vi "ATM.vi"() -> ()   [LabVIEW 2025]
uses:
  Controls/States.ctl
panel:
  in  "Enter":bool
  in  "User Input":string
  in  "Right Buttons":T1
  out "Right Menu":T2
  in  "Left Buttons":T1
  out "Left Menu":T2
  in  "Card Simulator":bool
  out "ATM Messages":string
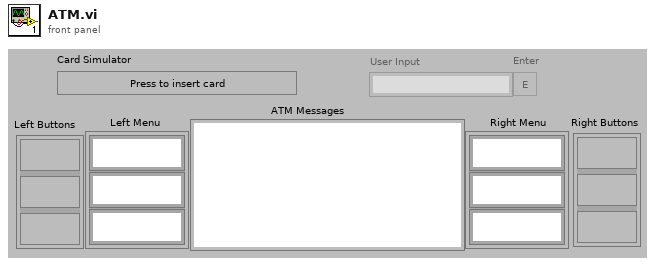
[diagram p1: front panel]
types:
  T1 = cluster{"Func Button":bool, "Func Button 2":bool, "Func Button 3":bool}
  T2 = cluster{"RFS String":string, "RFS String 2":string, "RFS String 3":string}
  T3 = typedef "States.ctl" = enum16{"Initialization", "Waiting For Instruction", "Card Inserted", "Identification", "Balance", "Deposit Message", "Deposit Complete", "Withdraw Message", "Withdraw Possible?", "Withdraw Complete", "Withdraw Failed", "Fast Cash", "Shutdown"}
  T4 = cluster{"Enter":refnum<vi>, "User Input":refnum<vi>, "Right Buttons":refnum<vi>, "Left Buttons":refnum<vi>, "Card Simulator":refnum<vi>, "Right Menu":refnum<vi>, "Left Menu":refnum<vi>, "ATM Messages":refnum<vi>}
  T5 = enum8{"Enabled", "Disabled", "Disabled and Grayed Out"}
  T6 = enum16{"Welcome", "Main Menu", "Account Verif Failed", "Session Terminate", "Deposit", "Deposit complete", "Withdrawal", "Withdrawal complete", "Withdrawal failed", "Balance Inquiry"}
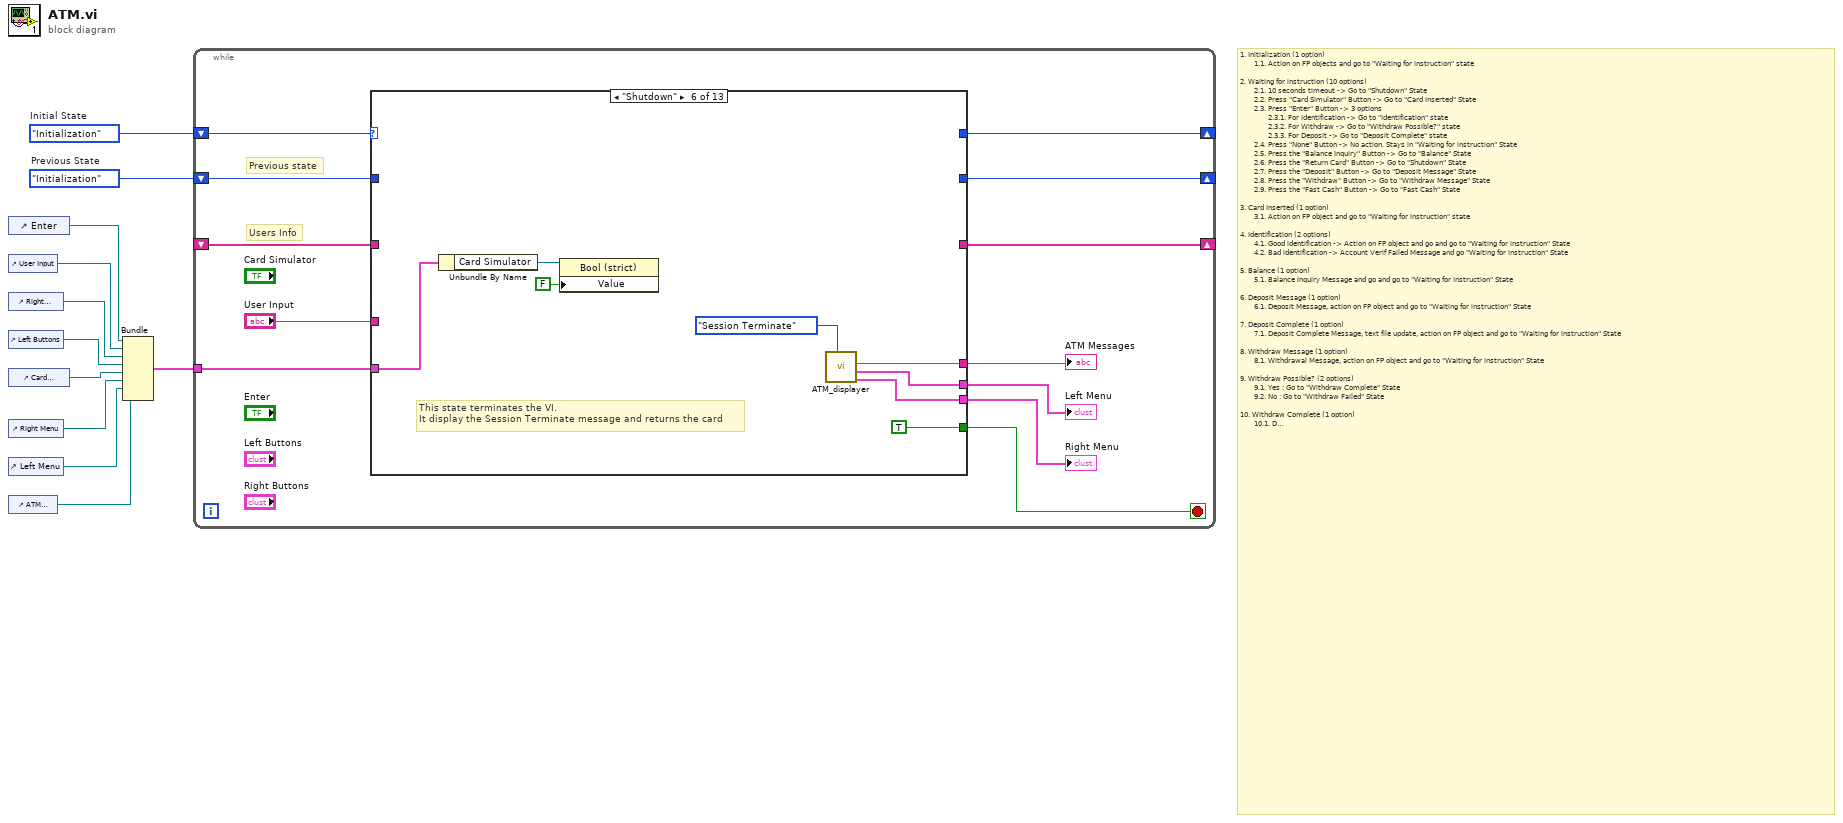
[diagram p0: block diagram]
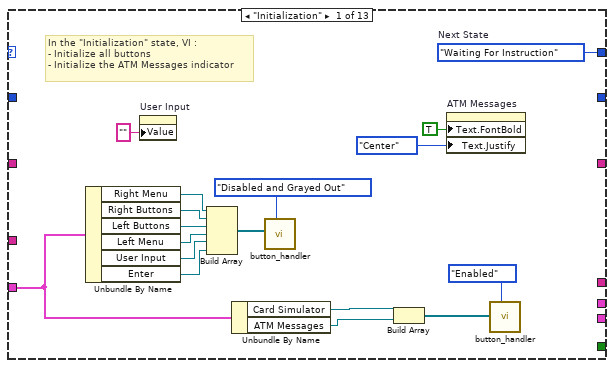
[diagram p2: hidden frame]
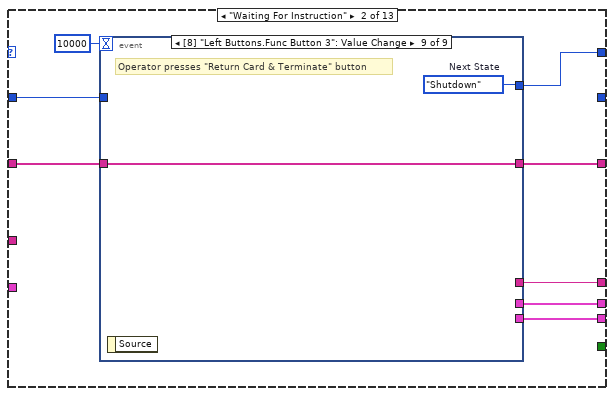
[diagram p3: hidden frame]
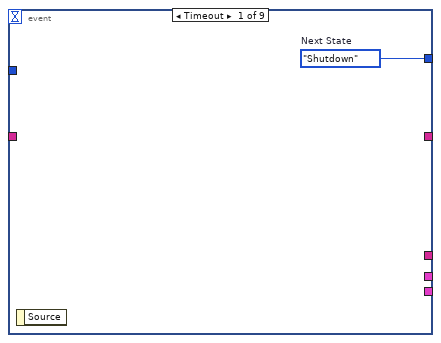
[diagram p4: hidden frame]
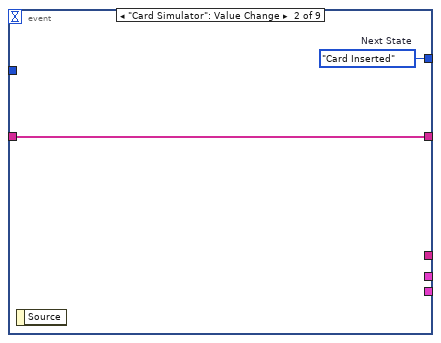
[diagram p5: hidden frame]
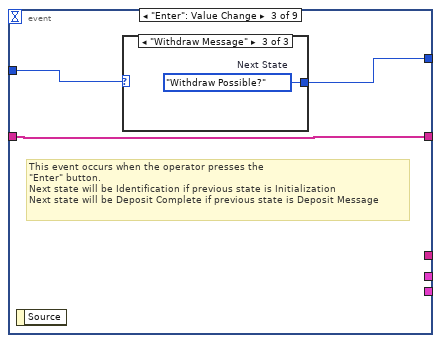
[diagram p6: hidden frame]
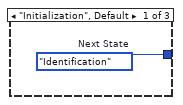
[diagram p7: hidden frame]
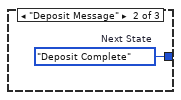
[diagram p8: hidden frame]
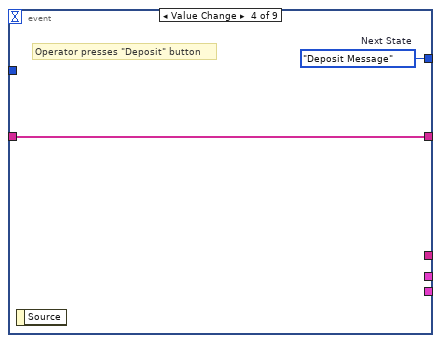
[diagram p9: hidden frame]
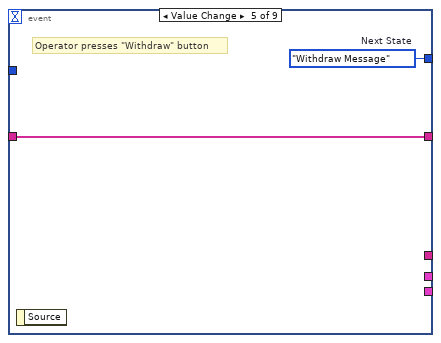
[diagram p10: hidden frame]
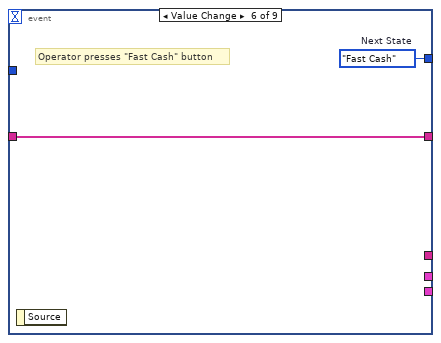
[diagram p11: hidden frame]
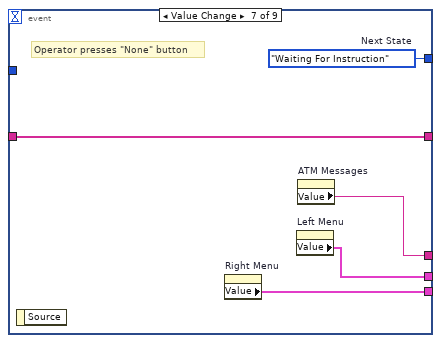
[diagram p12: hidden frame]
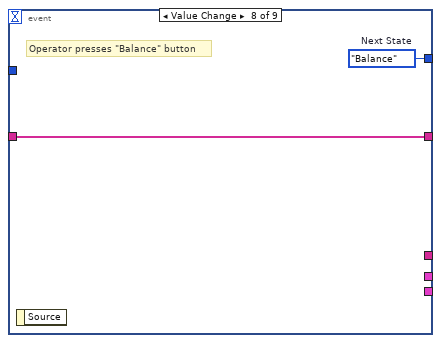
[diagram p13: hidden frame]
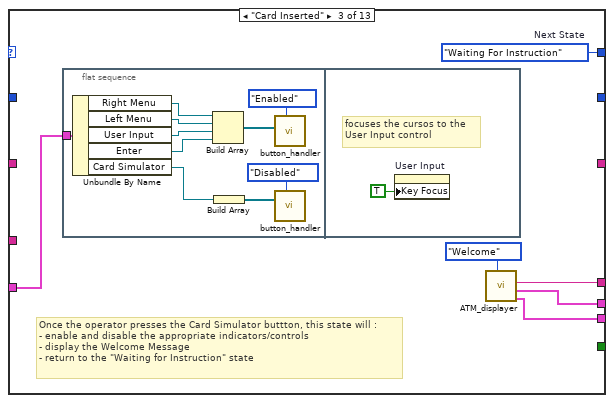
[diagram p14: hidden frame]
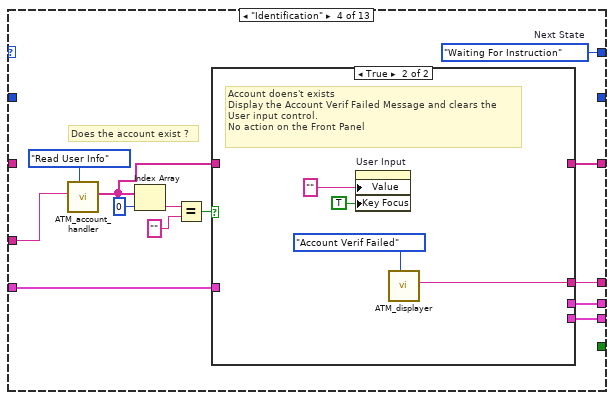
[diagram p15: hidden frame]
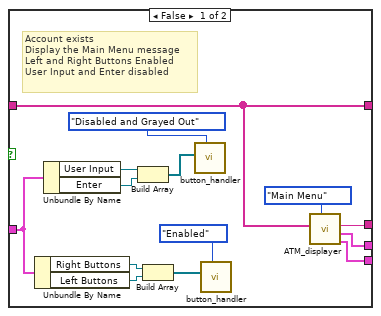
[diagram p16: hidden frame]
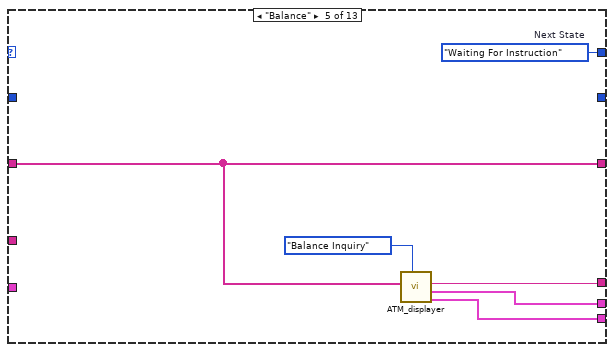
[diagram p17: hidden frame]
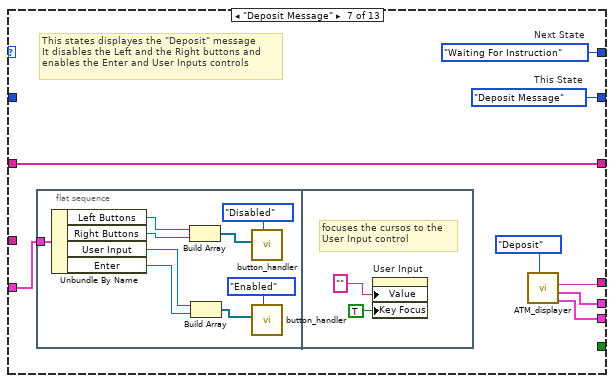
[diagram p18: hidden frame]
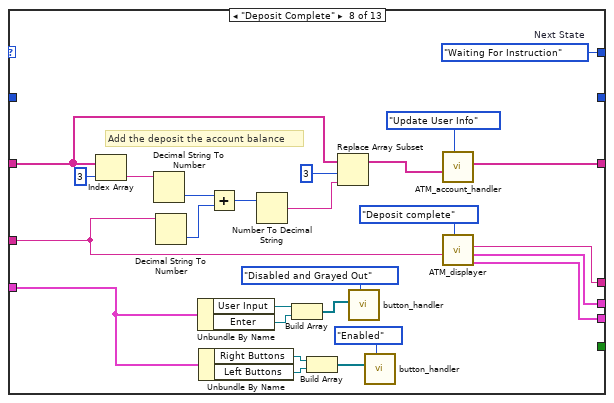
[diagram p19: hidden frame]
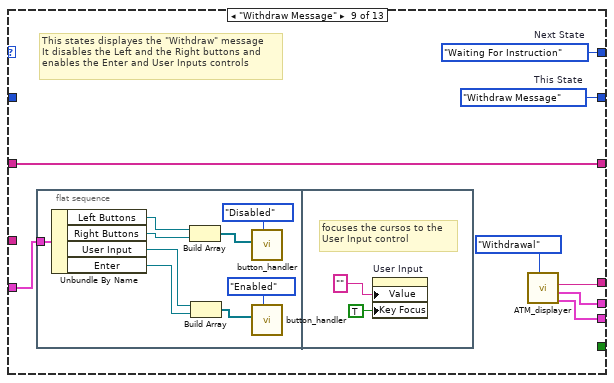
[diagram p20: hidden frame]
diagram:
  w1 = States."Initialization"  # Previous State
  w11 = States."Initialization"  # Initial State
  # "1. Initialization (1 option)\n       1.1. Action on FP objects and go to \"Waiting for instruction\" state\n\n2. Waiting for instruction (10 options)\n       2.1. 10 seconds timeout -> Go to \"Shutdown\" State\n       2.2. Press \"Card Simulator\" Button -> Go to \"Card Inserted\" State\n       2.3. Press \"Enter\" Button -> 3 options\n              2.3.1. For identification -> Go to \"Identification\" state  \n              2.3.2. For Withdraw -> Go to \"Withdraw Possible?\" state\n              2.3.3. For Deposit -> Go to \"Deposit Complete\" state\n       2.4. Press \"None\" Button -> No action. Stays in \"Waiting for instruction\" State\n       2.5. Press the \"Balance Inquiry\" Button -> Go to \"Balance\" State\n       2.6. Press the \"Return Card\" Button -> Go to \"Shutdown\" State\n       2.7. Press the \"Deposit\" Button -> Go to \"Deposit Message\" State\n       2.8. Press the \"Withdraw\" Button -> Go to \"Withdraw Message\" State\n       2.9. Press the \"Fast Cash\" Button -> Go to \"Fast Cash\" State\n\n3. Card Inserted (1 option)\n       3.1. Action on FP object and go to \"Waiting for instruction\" state\n\n4. Identification (2 options)\n       4.1. Good identification -> Action on FP object and go and go to \"Waiting for instruction\" State\n       4.2. Bad identification -> Account Verif Failed Message and go \"Waiting for instruction\" State\n\n5. Balance (1 option)\n       5.1. Balance Inquiry Message and go and go to \"Waiting for instruction\" State\n\n6. Deposit Message (1 option)\n       6.1. Deposit Message, action on FP object and go to \"Waiting for instruction\" State\n\n7. Deposit Complete (1 option)\n       7.1. Deposit Complete Message, text file update, action on FP object and go to \"Waiting for instruction\" State\n\n8. Withdraw Message (1 option)\n       8.1. Withdrawal Message, action on FP object and go to \"Waiting for instruction\" State\n\n9. Withdraw Possible? (2 options)\n       9.1. Yes : Go to \"Withdraw Complete\" State\n       9.2. No : Go to \"Withdraw Failed\" State\n\n10. Withdraw Complete (1 option)\n       10.1. Deposit Complete Message, text file update, action on FP object and go to \"Waiting for instructio\n\n11. Withdraw Failed (1 option)\n       11.1. Withdrawal Failed Message, action on FP object and go to \"Waiting for instructio\n\n12. Fast Cash (1 option)\n       12.1. Go to \"Withdrawal Possible?\" State\n\n13. Shutdown (1 option)\n       13.1. Session Terminate Message and Terminate Program"
  n1 = control-ref of="Enter"() -> (w10:refnum<vi>)
  n2 = control-ref of="User Input"() -> (w9:refnum<vi>)
  n3 = control-ref of="Right Buttons"() -> (w8:refnum<vi>)
  n4 = control-ref of="Left Buttons"() -> (w7:refnum<vi>)
  n5 = control-ref of="Card Simulator"() -> (w6:refnum<vi>)
  n6 = control-ref of="Right Menu"() -> (w5:refnum<vi>)
  n7 = control-ref of="Left Menu"() -> (w3:refnum<vi>)
  n8 = control-ref of="ATM Messages"() -> (w4:refnum<vi>)
  n9 = Bundle("Enter"=w10, "User Input"=w9, "Right Buttons"=w8, "Left Buttons"=w7, "Card Simulator"=w6, "Right Menu"=w5, "Left Menu"=w3, "ATM Messages"=w4) -> (w2:T4)  [unwired: 1 in]
  n10 = while {
    tunnel: w2 -> [w22]
    shift-right: [w21] -> _
    shift-left: w11 -> [w23]
    shift-right: [w15] -> _
    shift-left: _ -> [w14]
    shift-right: [w13] -> _
    shift-left: w1 -> [w12]
    stop <- w19 stop-if-true
    # "Previous state"
    # "Users Info"
    n11 = case shown="\"Shutdown\"" w23 {
      tunnel: w22 -> [w32 _ w73 w92 _ w129 w138 w156 w183 _ w230 w247 _]
      tunnel: [w25 w48 w75 w93 w123 _ w137 w176 w182 w199 w241 w256 w262] -> w21
      tunnel: [_ w46 w78 w96 w126 w133 w141 w154 w186 _ w229 w246 _] -> w20
      tunnel: [_ _ _ _ _ TRUE _ _ _ _ _ _ _] -> w19
      tunnel: [_ w45 w77 w95 w122 w132 w140 w179 w185 _ w244 w259 _] -> w18
      tunnel: [_ w44 w76 w94 w121 w131 w139 w178 w184 _ w243 w258 _] -> w17
      tunnel: "User Input" -> [_ _ _ w101 _ _ _ w155 _ w210 w223 _ _]
      tunnel: [_ w42 _ w90 w124 _ w136 w165 w181 w200 w239 w245 w261] -> w15
      tunnel: w14 -> [_ w43 _ _ w124 _ w136 w169 w181 w202 w228 w245 w261]
      tunnel: [_ _ _ _ _ _ w135 _ w180 w213 _ _ w260] -> w13
      tunnel: w12 -> [_ w41 _ _ _ _ _ _ _ w213 w226 _ _]
      frame "Initialization" {
        w25 = States."Waiting For Instruction"  # Next State
        # "In the \"Initialization\" state, VI :\n- Initialize all buttons\n- Initialize the ATM Messages indicator"
        n12 = Unbundle By Name(w32) -> ("Right Menu"=w40:refnum<vi>, "Right Buttons"=w39:refnum<vi>, "Left Buttons"=w38:refnum<vi>, "Left Menu"=w37:refnum<vi>, "User Input"=w36:refnum<vi>, "Enter"=w35:refnum<vi>)
        n13 = property on="User Input" class="Str"("Value"="" ("User Input")) -> ()  [unwired: 2 in, 2 out]
        n14 = Build Array(w40, w39, w38, w37, w36, w35) -> (w34:refnum<vi>[])
        n15 = Unbundle By Name(w32) -> ("Card Simulator"=w24:refnum<vi>, "ATM Messages"=w31:refnum<vi>)
        n16 = call "button_handler.vi"("Disabled"=T5."Disabled and Grayed Out", "reference"=w34) -> ()  [unwired: 10 in]
        n17 = Build Array(w24, w31) -> (w30:refnum<vi>[])
        n18 = property on="ATM Messages" class="Str"("Text.FontBold"=TRUE ("Text.Font:Bold"), "Text.Justify"=enum16{"Left", "Center", "Right"}."Center" ("Text.Justification")) -> ()  [unwired: 2 in, 2 out]
        n19 = call "button_handler.vi"("Disabled"=T5."Enabled", "reference"=w30) -> ()  [unwired: 10 in]
      }
      frame "Waiting For Instruction" {
        n20 = event shown="[8] \"Left Buttons.Func Button 3\": Value Change" {
          selector: _ -> [_ _ _ _ _ _ _ _ _]
          dyn-events: _ -> [_ _ _ _ _ _ _ _ _]
          timeout: 10000 -> [_ _ _ _ _ _ _ _ _]
          tunnel: [w49 w51 w54 w58 w60 w62 w68 w70 w72] -> w48
          tunnel: [_ _ _ _ _ _ w67 _ _] -> w46
          tunnel: [_ _ _ _ _ _ w66 _ _] -> w45
          tunnel: [_ _ _ _ _ _ w65 _ _] -> w44
          tunnel: w43 -> [_ w50 w53 w59 w61 w63 w64 w69 w71]
          tunnel: [_ w50 w53 w59 w61 w63 w64 w69 w71] -> w42
          tunnel: w41 -> [_ _ w52 _ _ _ _ _ _]
          event Timeout {
            w49 = States."Shutdown"  # Next State
            n21 = event-data() -> ()  [unwired: 1 in, 1 out]
          }
          event "Card Simulator": Value Change {
            w51 = States."Card Inserted"  # Next State
            n22 = event-data() -> ()  [unwired: 1 in, 1 out]
          }
          event "Enter": Value Change {
            # "This event occurs when the operator presses the\n\"Enter\" button.\nNext state will be Identification if previous state is Initialization\nNext state will be Deposit Complete if previous state is Deposit Message"
            n23 = event-data() -> ()  [unwired: 1 in, 1 out]
            n24 = case shown="\"Withdraw Message\"" w52 {
              tunnel: [w55 w56 w57] -> w54
              frame "Initialization", Default {
                w55 = States."Identification"  # Next State
              }
              frame "Deposit Message" {
                w56 = States."Deposit Complete"  # Next State
              }
              frame "Withdraw Message" {
                w57 = States."Withdraw Possible?"  # Next State
              }
            }
          }
          event "Right Buttons.Func Button": Value Change {
            w58 = States."Deposit Message"  # Next State
            # "Operator presses \"Deposit\" button"
            n25 = event-data() -> ()  [unwired: 1 in, 1 out]
          }
          event "Right Buttons.Func Button 2": Value Change {
            w60 = States."Withdraw Message"  # Next State
            # "Operator presses \"Withdraw\" button"
            n26 = event-data() -> ()  [unwired: 1 in, 1 out]
          }
          event "Right Buttons.Func Button 3": Value Change {
            w62 = States."Fast Cash"  # Next State
            # "Operator presses \"Fast Cash\" button"
            n27 = event-data() -> ()  [unwired: 1 in, 1 out]
          }
          event "Left Buttons.Func Button": Value Change {
            w68 = States."Waiting For Instruction"  # Next State
            # "Operator presses \"None\" button"
            n28 = event-data() -> ()  [unwired: 1 in, 1 out]
            n29 = property on="Right Menu" class="Clust (strict)"() -> ("Value"=w65:T2)  [unwired: 2 in, 2 out]
            n30 = property on="Left Menu" class="Clust (strict)"() -> ("Value"=w66:T2)  [unwired: 2 in, 2 out]
            n31 = property on="ATM Messages" class="Str"() -> ("Value"=w67:string)  [unwired: 2 in, 2 out]
          }
          event "Left Buttons.Func Button 2": Value Change {
            w70 = States."Balance"  # Next State
            # "Operator presses \"Balance\" button"
            n32 = event-data() -> ()  [unwired: 1 in, 1 out]
          }
          event "Left Buttons.Func Button 3": Value Change {
            w72 = States."Shutdown"  # Next State
            # "Operator presses \"Return Card & Terminate\" button"
            n33 = event-data() -> ()  [unwired: 1 in, 1 out]
          }
        }
      }
      frame "Card Inserted" {
        w75 = States."Waiting For Instruction"  # Next State
        # "Once the operator presses the Card Simulator buttton, this state will :\n- enable and disable the appropriate indicators/controls\n- display the Welcome Message\n- return to the \"Waiting for Instruction\" state"
        n34 = flat-sequence {
          tunnel: w73 -> [w88]
          frame #0 {
            n35 = Unbundle By Name(w88) -> ("Right Menu"=w87:refnum<vi>, "Left Menu"=w86:refnum<vi>, "User Input"=w85:refnum<vi>, "Enter"=w84:refnum<vi>, "Card Simulator"=w83:refnum<vi>)
            n36 = Build Array(w87, w86, w85, w84) -> (w82:refnum<vi>[])
            n37 = Build Array(w83) -> (w81:refnum<vi>[])
            n38 = call "button_handler.vi"("Disabled"=T5."Enabled", "reference"=w82) -> ()  [unwired: 10 in]
            n39 = call "button_handler.vi"("Disabled"=T5."Disabled", "reference"=w81) -> ()  [unwired: 10 in]
          }
          frame #1 {
            # "focuses the cursos to the \nUser Input control"
            n40 = property on="User Input" class="Str"("Key Focus"=TRUE) -> ()  [unwired: 2 in, 2 out]
          }
        }
        n41 = call "ATM_displayer.vi"("Message"=T6."Welcome") -> ("Right Menu"=w76:cluster{string, string, string}, "Left Menu"=w77:cluster{string, string, string}, "Message display"=w78:string)  [unwired: 8 in]
      }
      frame "Identification" {
        w93 = States."Waiting For Instruction"  # Next State
        # "Does the account exist ?"
        n42 = call "ATM_account_handler.vi"("Action"=enum16{"Read User Info", "Update User Info"}."Read User Info", "User Input (for read)"=w101) -> ("Users info"=w91:string[])  [unwired: 9 in]
        n43 = Index Array(array=w91, index=0) -> (element=w99:string)
        n44 = Equal?(x=w99, y="") -> (x = y?=w97:bool)
        n45 = case shown="True" w97 {
          tunnel: [w115 w119] -> w96
          tunnel: [w114 _] -> w95
          tunnel: [w113 _] -> w94
          tunnel: w92 -> [w108 _]
          tunnel: w91 -> [w103 _]
          tunnel: [w103 _] -> w90
          frame False {
            # "Account exists\nDisplay the Main Menu message\nLeft and Right Buttons Enabled\nUser Input and Enter disabled"
            n46 = Unbundle By Name(w108) -> ("Right Buttons"=w107:refnum<vi>, "Left Buttons"=w106:refnum<vi>)
            n47 = Unbundle By Name(w108) -> ("User Input"=w111:refnum<vi>, "Enter"=w110:refnum<vi>)
            n48 = Build Array(w111, w110) -> (w109:refnum<vi>[])
            n49 = Build Array(w107, w106) -> (w104:refnum<vi>[])
            n50 = call "button_handler.vi"("Disabled"=T5."Disabled and Grayed Out", "reference"=w109) -> ()  [unwired: 10 in]
            n51 = call "button_handler.vi"("Disabled"=T5."Enabled", "reference"=w104) -> ()  [unwired: 10 in]
            n52 = call "ATM_displayer.vi"("Message"=T6."Main Menu", "Users Info"=w103) -> ("Right Menu"=w113:cluster{string, string, string}, "Left Menu"=w114:cluster{string, string, string}, "Message display"=w115:string)  [unwired: 7 in]
          }
          frame True {
            # "Account doens't exists\nDisplay the Account Verif Failed Message and clears the\nUser input control.\nNo action on the Front Panel"
            n53 = property on="User Input" class="Str"("Value"="" ("User Input"), "Key Focus"=TRUE) -> ()  [unwired: 2 in, 2 out]
            n54 = call "ATM_displayer.vi"("Message"=T6."Account Verif Failed") -> ("Message display"=w119:string)  [unwired: 8 in, 2 out]
          }
        }
      }
      frame "Balance" {
        w123 = States."Waiting For Instruction"  # Next State
        n55 = call "ATM_displayer.vi"("Message"=T6."Balance Inquiry", "Users Info"=w124) -> ("Right Menu"=w121:cluster{string, string, string}, "Left Menu"=w122:cluster{string, string, string}, "Message display"=w126:string)  [unwired: 7 in]
      }
      frame "Shutdown" {
        # "This state terminates the VI.\nIt display the Session Terminate message and returns the card"
        n56 = Unbundle By Name(w129) -> ("Card Simulator"=w128:refnum<vi>)
        n57 = property class="Bool (strict)"(reference=w128, "Value"=FALSE) -> ()  [unwired: 1 in, 2 out]
        n58 = call "ATM_displayer.vi"("Message"=T6."Session Terminate") -> ("Right Menu"=w131:cluster{string, string, string}, "Left Menu"=w132:cluster{string, string, string}, "Message display"=w133:string)  [unwired: 8 in]
      }
      frame "Deposit Message" {
        w135 = States."Deposit Message"  # This State
        w137 = States."Waiting For Instruction"  # Next State
        # "This states displayes the \"Deposit\" message\nIt disables the Left and the Right buttons and \nenables the Enter and User Inputs controls"
        n59 = flat-sequence {
          tunnel: w138 -> [w146]
          frame #0 {
            n60 = Unbundle By Name(w146) -> ("Left Buttons"=w151:refnum<vi>, "Right Buttons"=w150:refnum<vi>, "User Input"=w145:refnum<vi>, "Enter"=w144:refnum<vi>)
            n61 = Build Array(w151, w150) -> (w149:refnum<vi>[])
            n62 = Build Array(w145, w144) -> (w143:refnum<vi>[])
            n63 = call "button_handler.vi"("Disabled"=T5."Disabled", "reference"=w149) -> ()  [unwired: 10 in]
            n64 = call "button_handler.vi"("Disabled"=T5."Enabled", "reference"=w143) -> ()  [unwired: 10 in]
          }
          frame #1 {
            # "focuses the cursos to the \nUser Input control"
            n65 = property on="User Input" class="Str"("Value"="" ("User Input"), "Key Focus"=TRUE) -> ()  [unwired: 2 in, 2 out]
          }
        }
        n66 = call "ATM_displayer.vi"("Message"=T6."Deposit") -> ("Right Menu"=w139:cluster{string, string, string}, "Left Menu"=w140:cluster{string, string, string}, "Message display"=w141:string)  [unwired: 8 in]
      }
      frame "Deposit Complete" {
        w176 = States."Waiting For Instruction"  # Next State
        # "Add the deposit the account balance"
        n67 = Index Array(array=w169, index=3) -> (element=w174:string)
        n68 = Decimal String To Number(string=w174) -> (number=w173:i32)  [unwired: 2 in, 1 out]
        n69 = Decimal String To Number(string=w155) -> (number=w172:i32)  [unwired: 2 in, 1 out]
        n70 = Unbundle By Name(w156) -> ("User Input"=w164:refnum<vi>, "Enter"=w163:refnum<vi>)
        n71 = Unbundle By Name(w156) -> ("Right Buttons"=w160:refnum<vi>, "Left Buttons"=w159:refnum<vi>)
        n72 = Add(x=w173, y=w172) -> (x+y=w171:i32)
        n73 = Number To Decimal String(number=w171) -> (decimal integer string=w167:string)  [unwired: 1 in]
        n74 = Build Array(w164, w163) -> (w162:refnum<vi>[])
        n75 = Build Array(w160, w159) -> (w158:refnum<vi>[])
        n76 = Replace Array Subset(array=w169, new element=w167, index=3) -> (w166:string[])
        n77 = call "button_handler.vi"("Disabled"=T5."Disabled and Grayed Out", "reference"=w162) -> ()  [unwired: 10 in]
        n78 = call "button_handler.vi"("Disabled"=T5."Enabled", "reference"=w158) -> ()  [unwired: 10 in]
        n79 = call "ATM_account_handler.vi"("Action"=enum16{"Read User Info", "Update User Info"}."Update User Info", "Users info (for update)"=w166) -> ("Users info"=w165:string[])  [unwired: 9 in]
        n80 = call "ATM_displayer.vi"("Message"=T6."Deposit complete", "Amount"=w155) -> ("Right Menu"=w178:cluster{string, string, string}, "Left Menu"=w179:cluster{string, string, string}, "Message display"=w154:string)  [unwired: 7 in]
      }
      frame "Withdraw Message" {
        w180 = States."Withdraw Message"  # This State
        w182 = States."Waiting For Instruction"  # Next State
        # "This states displayes the \"Withdraw\" message\nIt disables the Left and the Right buttons and \nenables the Enter and User Inputs controls"
        n81 = flat-sequence {
          tunnel: w183 -> [w191]
          frame #0 {
            n82 = Unbundle By Name(w191) -> ("Left Buttons"=w196:refnum<vi>, "Right Buttons"=w195:refnum<vi>, "User Input"=w190:refnum<vi>, "Enter"=w189:refnum<vi>)
            n83 = Build Array(w196, w195) -> (w194:refnum<vi>[])
            n84 = Build Array(w190, w189) -> (w188:refnum<vi>[])
            n85 = call "button_handler.vi"("Disabled"=T5."Disabled", "reference"=w194) -> ()  [unwired: 10 in]
            n86 = call "button_handler.vi"("Disabled"=T5."Enabled", "reference"=w188) -> ()  [unwired: 10 in]
          }
          frame #1 {
            # "focuses the cursos to the \nUser Input control"
            n87 = property on="User Input" class="Str"("Value"="" ("User Input"), "Key Focus"=TRUE) -> ()  [unwired: 2 in, 2 out]
          }
        }
        n88 = call "ATM_displayer.vi"("Message"=T6."Withdrawal") -> ("Right Menu"=w184:cluster{string, string, string}, "Left Menu"=w185:cluster{string, string, string}, "Message display"=w186:string)  [unwired: 8 in]
      }
      frame "Withdraw Possible?" {
        # "Is Previous state \"Fast Cash\" ?"
        # "This case will determine if account has enough to perform a Withdraw.\nIf the previous state is \"Fast Cash\", the code will use 50 to perform the substration (balance - 50) \nIf not, the code will use User Input to perform the substraction (balance - User Input)"
        n89 = Decimal String To Number(string=w210) -> (number=w209:i32)  [unwired: 2 in, 1 out]
        n90 = Equal?(x=w213, y=States."Fast Cash") -> (x = y?=w208:bool)
        n91 = Select(t=50, s=w208, f=w209) -> (s? t:f=w204:i32)
        n92 = Index Array(array=w202, index=3) -> (element=w206:string)
        n93 = Decimal String To Number(string=w206) -> (number=w205:i32)  [unwired: 2 in, 1 out]
        n94 = Subtract(x=w205, y=w204) -> (x-y=w201:i32)
        n95 = Greater Or Equal To 0?(x=w201) -> (x >= 0?=w203:bool)
        n96 = case shown="False" w203 {
          tunnel: w202 -> [w215 w221]
          tunnel: w201 -> [_ w219]
          tunnel: [w215 w217] -> w200
          tunnel: [w214 w216] -> w199
          frame False {
            w214 = States."Withdraw Failed"  # Next State
            # "Not enough money"
          }
          frame True {
            w216 = States."Withdraw Complete"  # Next State
            # "Enough Money"
            n97 = Number To Decimal String(number=w219) -> (decimal integer string=w218:string)  [unwired: 1 in]
            n98 = Insert Into Array(array=w221, index=3, new element=w218) -> (w217:string[])
          }
        }
      }
      frame "Withdraw Complete" {
        w241 = States."Waiting For Instruction"  # Next State
        # "This case will display the \"Withdrawal Complete\" message, \nupdate the \"ATM accounts\" file with the new balance and \ndisable/enable the FP buttons needed"
        # "Is Previous state \"Fast Cash\" ?"
        n99 = Equal?(x=w226, y=States."Fast Cash") -> (x = y?=w225:bool)
        n100 = Unbundle By Name(w230) -> ("User Input"=w238:refnum<vi>, "Enter"=w237:refnum<vi>)
        n101 = Unbundle By Name(w230) -> ("Right Buttons"=w234:refnum<vi>, "Left Buttons"=w233:refnum<vi>)
        n102 = Select(t="50", s=w225, f=w223) -> (s? t:f=w222:string)
        n103 = Build Array(w238, w237) -> (w236:refnum<vi>[])
        n104 = Build Array(w234, w233) -> (w232:refnum<vi>[])
        n105 = call "button_handler.vi"("Disabled"=T5."Disabled and Grayed Out", "reference"=w236) -> ()  [unwired: 10 in]
        n106 = call "button_handler.vi"("Disabled"=T5."Enabled", "reference"=w232) -> ()  [unwired: 10 in]
        n107 = call "ATM_account_handler.vi"("Action"=enum16{"Read User Info", "Update User Info"}."Update User Info", "Users info (for update)"=w228) -> ("Users info"=w239:string[])  [unwired: 9 in]
        n108 = call "ATM_displayer.vi"("Message"=T6."Withdrawal complete", "Amount"=w222) -> ("Right Menu"=w243:cluster{string, string, string}, "Left Menu"=w244:cluster{string, string, string}, "Message display"=w229:string)  [unwired: 7 in]
      }
      frame "Withdraw Failed" {
        w256 = States."Waiting For Instruction"  # Next State
        # "This case will display the \"Withdrawal Failed\" message and\ndisable/enable the FP buttons needed"
        n109 = Unbundle By Name(w247) -> ("User Input"=w255:refnum<vi>, "Enter"=w254:refnum<vi>)
        n110 = Unbundle By Name(w247) -> ("Right Buttons"=w251:refnum<vi>, "Left Buttons"=w250:refnum<vi>)
        n111 = Build Array(w255, w254) -> (w253:refnum<vi>[])
        n112 = Build Array(w251, w250) -> (w249:refnum<vi>[])
        n113 = call "button_handler.vi"("Disabled"=T5."Disabled and Grayed Out", "reference"=w253) -> ()  [unwired: 10 in]
        n114 = call "button_handler.vi"("Disabled"=T5."Enabled", "reference"=w249) -> ()  [unwired: 10 in]
        n115 = call "ATM_displayer.vi"("Message"=T6."Withdrawal failed") -> ("Right Menu"=w258:cluster{string, string, string}, "Left Menu"=w259:cluster{string, string, string}, "Message display"=w246:string)  [unwired: 8 in]
      }
      frame "Fast Cash" {
        w260 = States."Fast Cash"  # This State
        w262 = States."Withdraw Possible?"  # Next State
        # "This case occurs if the operator has pressed the \"Fast Cash\" action button."
      }
    }
    "ATM Messages" <- w20
    "Left Menu" <- w18
    "Right Menu" <- w17
  }
